vi "terminate.vi"(8 "error in (no error)":errorcluster, 11 "GenericImageAssembler in":refnum<class "GenericImageAssembler.lvclass">) -> (0 "error out":errorcluster, 3 "GenericImageAssembler out":refnum<class "GenericImageAssembler.lvclass">)   [LabVIEW 2010]
uses:
  class_data.vi
  GenericImageAssembler.lvclass
  common/classes/Image/Image/Image.lvclass
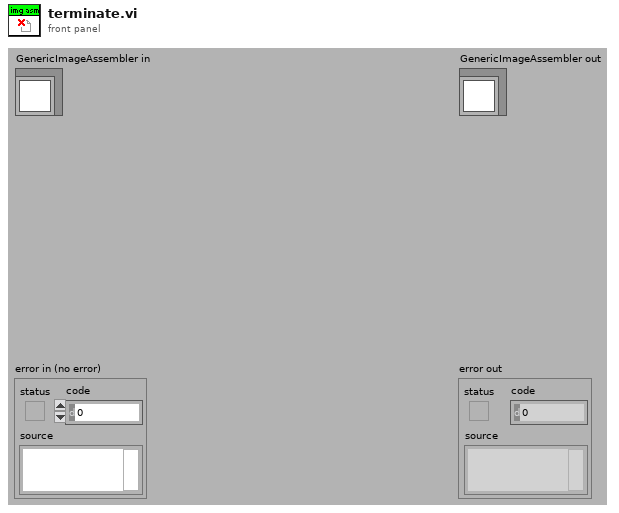
[diagram p1: front panel]
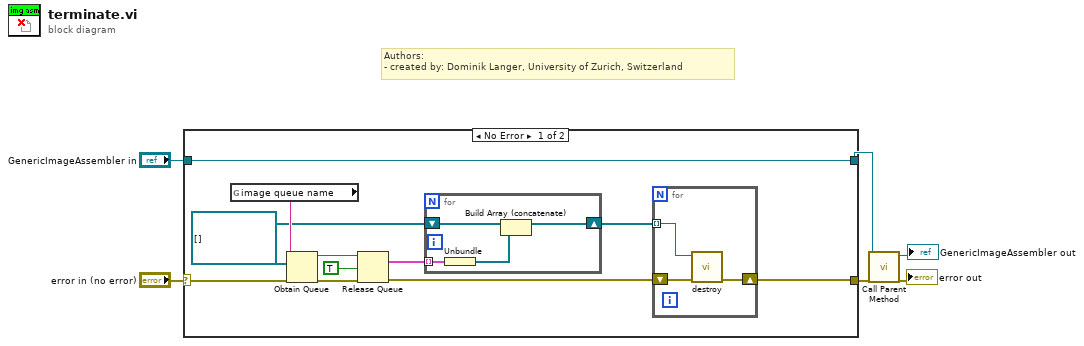
[diagram p0: block diagram]
diagram:
  # "Authors: \n- created by: Dominik Langer, University of Zurich, Switzerland"
  n1 = case shown="No Error" "error in (no error)" {
    selector: "error in (no error)" -> [w14 w26]
    tunnel: [w9 w26] -> w4
    tunnel: [w8 w25] -> w2
    tunnel: "GenericImageAssembler in" -> [w8 w25]
    frame No Error {
      w10 = refnum<class "Image.lvclass">[] []
      n2 = global read "class_data.vi" "image queue name"() -> (w12:string)
      n3 = Obtain Queue(name (unnamed)=w12, element data type=w10, error in (no error)=w14) -> (queue out=w16:refnum<queue>, error out=w17:errorcluster)  [unwired: 2 in, 1 out]
      n4 = Release Queue(queue=w16, force destroy? (F)=TRUE, error in (no error)=w17) -> (remaining elements=w11:cluster{refnum<class "Image.lvclass">[]}[], error out=w13:errorcluster)  [unwired: 1 out]
      n5 = for {
        tunnel: w11 -> [w21] mode=indexing
        shift-right: [w18] -> w7
        shift-left: w10 -> [w20]
        n6 = Unbundle(w21) -> (w19:refnum<class "Image.lvclass">[])
        n7 = Build Array (concatenate)(w20, w19) -> (w18:refnum<class "Image.lvclass">[])
      }
      n8 = for {
        tunnel: w7 -> [w24] mode=indexing
        shift-right: [w22] -> w9
        shift-left: w13 -> [w23]
        n9 = call-dynamic "destroy.vi"("error in (no error)"=w23, "Image in"=w24) -> ("error out"=w22:errorcluster)  [unwired: 9 out]
      }
    }
    frame Error {
    }
  }
  n10 = call-parent "Call Parent Method"("error in (no error)"=w4, "GenericPlugin in"=w2) -> ("error out"=→"error out":errorcluster, "GenericPlugin out"=→"GenericImageAssembler out":refnum<class "GenericImageAssembler.lvclass">)  [unwired: 8 out]
